vi "processState.vi"(8 "error in (no error)":errorcluster, 11 "guiTemplates in":refnum<class "stillnessHelper.lvclass">) -> (0 "error out":errorcluster, 1 "Options":string[](array[string]), 2 "States":string(combo), 3 "guiTemplates out":refnum<class "stillnessHelper.lvclass">, 5 "Timeout":i32)   [LabVIEW 2022 SP3, in "stillnessHelper.lvclass"]
uses:
  stillnessHelper.lvclass
  stillnessHelper.lvclass/stillnessHelper.ctl
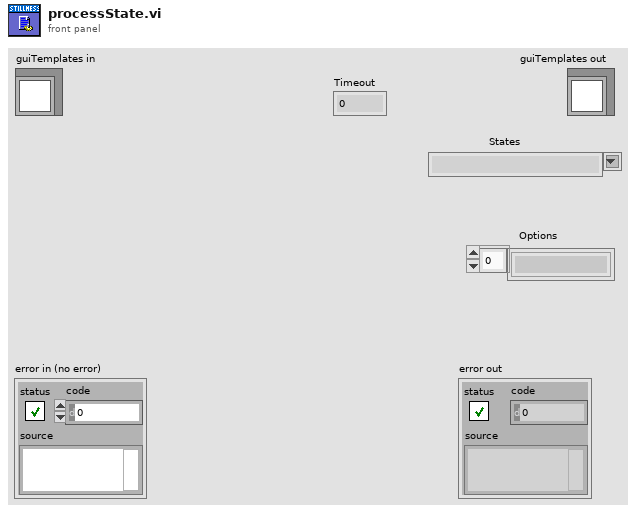
[diagram p1: front panel]
types:
  T1 = typedef "guiTemplates.lvclass/statesWithOptions.ctl" = cluster{"States":string, "Options":string[]}
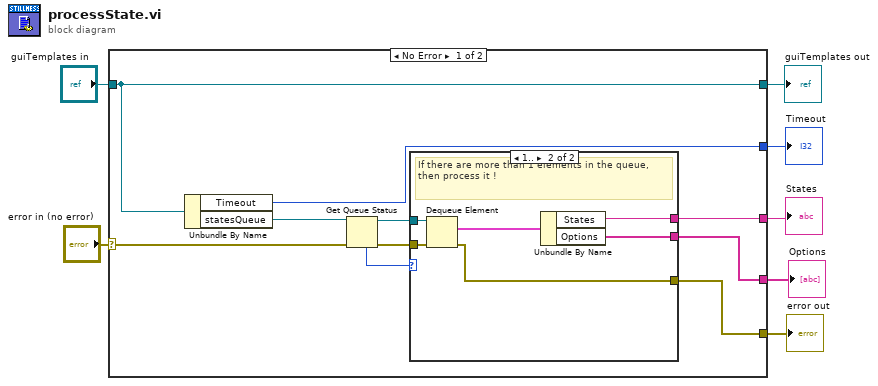
[diagram p0: block diagram]
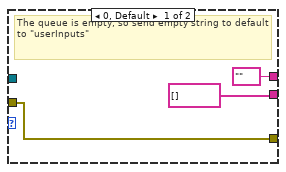
[diagram p2: hidden frame]
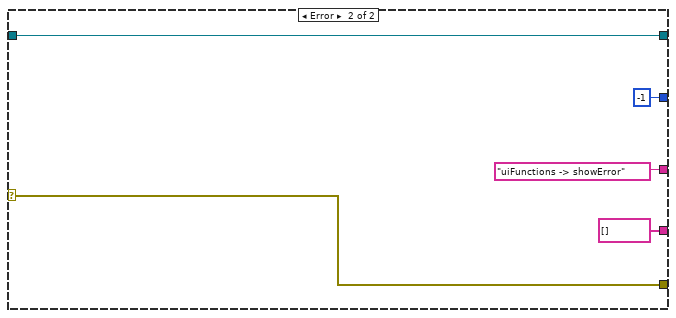
[diagram p3: hidden frame]
diagram:
  n1 = case shown="No Error" "error in (no error)" {
    selector: "error in (no error)" -> [w10 w30]
    tunnel: [w9 w30] -> w6
    tunnel: [w17 w31] -> w4
    tunnel: "guiTemplates in" -> [w17 w31]
    tunnel: [w12 "uiFunctions -> showError" ("States")] -> w3
    tunnel: [w11 string[] [] ("Options")] -> w2
    tunnel: [w8 -1 ("Timeout")] -> w1
    frame No Error {
      n2 = Unbundle By Name(w17) -> ("Timeout"=w8:i32, "statesQueue"=w13:refnum<queue>)
      n3 = Get Queue Status(queue=w13, error in (no error)=w10) -> (queue out=w15:refnum<queue>, error out=w16:errorcluster, # elements in queue=w14:i32)  [unwired: 1 in, 5 out]
      n4 = case shown="1.." w14 {
        tunnel: w15 -> [_ w26]
        tunnel: w16 -> [w19 w25]
        tunnel: [string[] [] ("Options") w23] -> w11
        tunnel: [w19 w22] -> w9
        tunnel: ["" ("States") w21] -> w12
        frame 0, Default {
          # "The queue is empty, so send empty string to default to \"userInputs\""
        }
        frame 1.. {
          # "If there are more than 1 elements in the queue, then process it !"
          n5 = Dequeue Element(queue=w26, error in (no error)=w25) -> (element=w24:T1, error out=w22:errorcluster)  [unwired: 1 in, 2 out]
          n6 = Unbundle By Name(w24) -> ("States"=w21:string, "Options"=w23:string[])
        }
      }
    }
    frame Error {
    }
  }
  "error out" <- w6
  "guiTemplates out" <- w4
  "States" <- w3
  "Options" <- w2
  "Timeout" <- w1
